vi "l_matr_v0.vi"() -> ()   [LabVIEW 2009]
panel:
  in  "Date":u8(slide) scale=0.0..31.0
  out "Array 2":bool[](array[boolean])=[FALSE, FALSE, FALSE, TRUE, TRUE, FALSE, FALSE, FALSE]
  in  "Linia":u8(slide) scale=0.0..6.0
  in  "Iesire":bool
  in  "Automat":bool=TRUE
  out "Array":bool[](array[boolean])=[FALSE, FALSE, FALSE, TRUE, TRUE, FALSE, FALSE, FALSE]
  # "Manual"
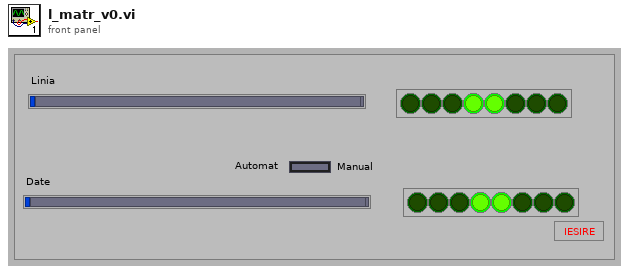
[diagram p1: front panel]
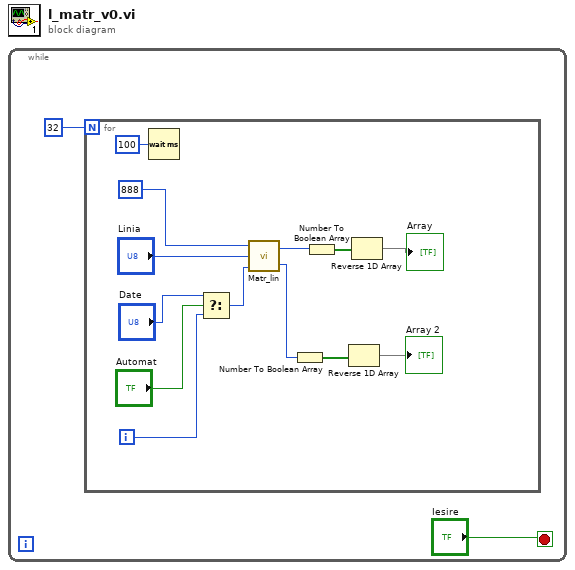
[diagram p0: block diagram]
diagram:
  n1 = while {
    stop <- "Iesire" stop-if-true
    n2 = for {
      N: 32 -> [_]
      i -> [w8]
      n3 = Wait (ms)(milliseconds to wait=u32 100) -> ()  [unwired: 1 out]
      n4 = Select(t="Date", s="Automat", f=w8) -> (s? t:f=w6:i32)
      n5 = call "Matr_lin.vi"("Date"=w6, "Linia"="Linia", "Adresa"=888) -> ("Numeric"=w4:u8, "D0-D7"=w5:u8)
      n6 = Number To Boolean Array(number=w4) -> (Boolean array=w11:bool[])
      n7 = Number To Boolean Array(number=w5) -> (Boolean array=w15:bool[])
      n8 = Reverse 1D Array(array=w11) -> (reversed array=→"Array 2":bool[])
      n9 = Reverse 1D Array(array=w15) -> (reversed array=→"Array":bool[])
    }
  }
